vi "Open Panel.vi"(8 "error in (no error)":errorcluster, 11 "[MV] Key Certify in":refnum<class "[MV] Key Certify.lvclass">) -> (0 "error out":errorcluster, 3 "[MV] Key Certify out":refnum<class "[MV] Key Certify.lvclass">)   [LabVIEW 2023, in "[MV] Key Certify.lvlib" / "[MV] Key Certify.lvclass"]
uses:
  [MV] Key Certify.lvclass
  [MV] Key Certify.lvclass/[MV] Key Certify.ctl
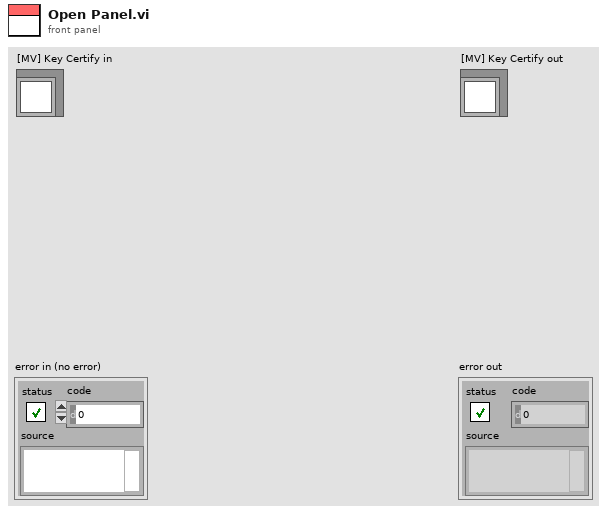
[diagram p1: front panel]
types:
  T1 = enum32{"Invalid", "Standard", "Closed", "Hidden", "Minimized", "Maximized"}
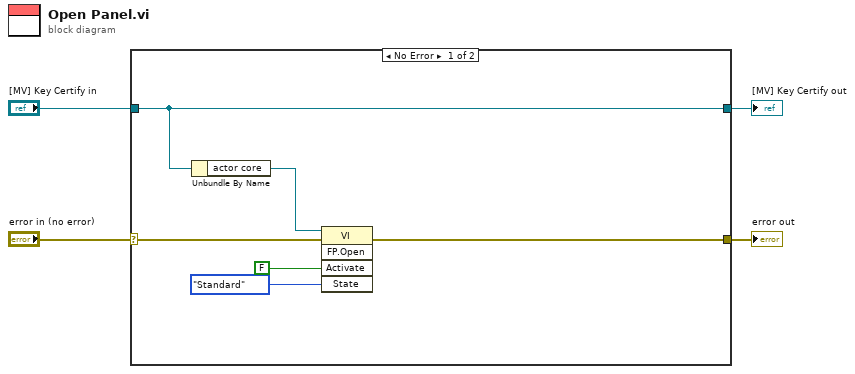
[diagram p0: block diagram]
diagram:
  n1 = case shown="No Error" "error in (no error)" {
    selector: "error in (no error)" -> [w10 w12]
    tunnel: [w8 w12] -> w3
    tunnel: [w9 w11] -> w1
    tunnel: "[MV] Key Certify in" -> [w9 w11]
    frame No Error {
      n2 = Unbundle By Name(w9) -> ("actor core"=w7:refnum<vi>)
      n3 = invoke class="VI" method="FP.Open"(reference=w7, error in=w10, "Activate"=FALSE ("Activate?"), "State"=T1."Standard") -> (error out=w8:errorcluster)  [unwired: 1 in, 4 out]
    }
    frame Error {
    }
  }
  "error out" <- w3
  "[MV] Key Certify out" <- w1
